vi "Drop Waypoint.vi"(1 "TA Speed":dbl, 2 "TA GPS":cluster{"X pos":i32, "Y pos":i32, "Heading":dbl}={"X pos"=250, "Y pos"=250, "Heading"=0.0}, 3 "Our GPS":cluster{"X pos":i32, "Y pos":i32, "Heading":dbl}={"X pos"=250, "Y pos"=250, "Heading"=0.0}) -> (0 "Output Waypoint":T1={"Type"=enum."Start", "X"=250, "Y"=250, "Speed"=0, "Behaviors"=enum."Open Water Transit"})   [LabVIEW 2014]
panel:
  in  "Waypoint seed":T1={"Type"=enum."Start", "X"=250, "Y"=250, "Speed"=0, "Behaviors"=enum."Open Water Transit"}
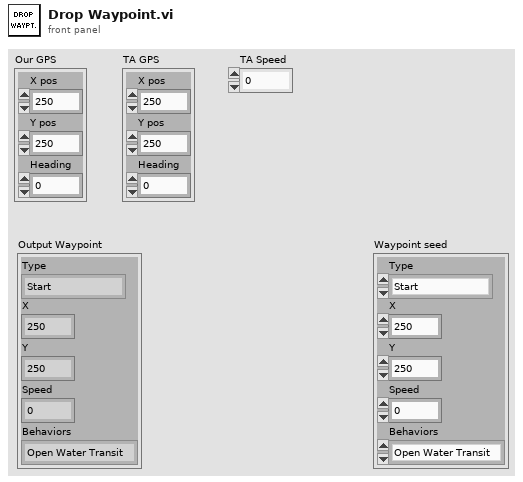
[diagram p1: front panel]
types:
  T1 = cluster{"Type":enum16{"Start", "Waypoint", "End"}, "X":i32, "Y":i32, "Speed":i32, "Behaviors":enum16{"Open Water Transit", "P-Wall Follow", "S-Wall Follow", "Dock", "Chase"}}
  T2 = enum16{"Open Water Transit", "P-Wall Follow", "S-Wall Follow", "Dock", "Chase"}
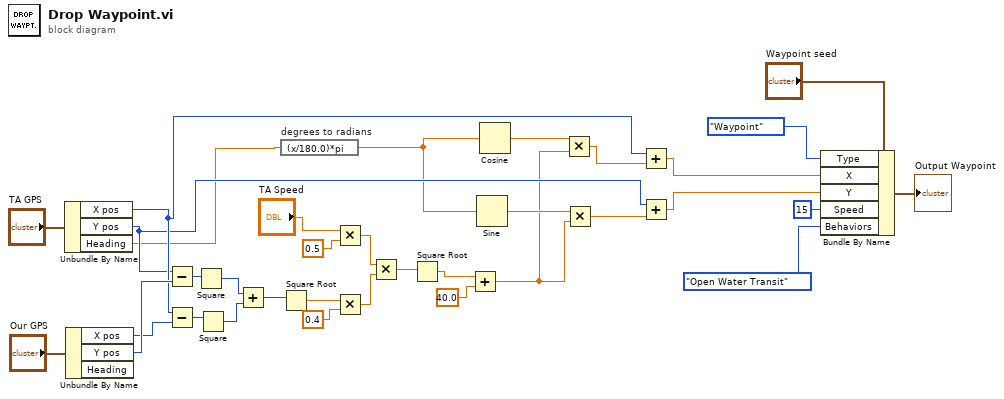
[diagram p0: block diagram]
diagram:
  n1 = Unbundle By Name("TA GPS") -> ("X pos"=w12:i32, "Y pos"=w10:i32, "Heading"=w2:dbl)
  n2 = Unbundle By Name("Our GPS") -> ("X pos"=w27:i32, "Y pos"=w28:i32)  [unwired: 1 out]
  n3 = Subtract(x=w10, y=w28) -> (x-y=w26:i32)
  n4 = Subtract(x=w12, y=w27) -> (x-y=w25:i32)
  n5 = Square(x=w26) -> (x^2=w23:i32)
  n6 = Square(x=w25) -> (x^2=w22:i32)
  n7 = Add(x=w23, y=w22) -> (x+y=w24:i32)
  n8 = expression code="(x/180.0)*pi" "degrees to radians"(w2) -> (w1:dbl)
  n9 = Square Root(x=w24) -> (sqrt(x)=w21:dbl)
  n10 = Multiply(x="TA Speed", y=0.5) -> (x*y=w3:dbl)
  n11 = Multiply(x=w21, y=0.4) -> (x*y=w18:dbl)
  n12 = Multiply(x=w3, y=w18) -> (x*y=w6:dbl)
  n13 = Square Root(x=w6) -> (sqrt(x)=w5:dbl)
  n14 = Add(x=w5, y=40.0) -> (x+y=w8:dbl)
  n15 = Sine(x=w1) -> (sin(x)=w16:dbl)
  n16 = Cosine(x=w1) -> (cos(x)=w15:dbl)
  n17 = Multiply(x=w15, y=w8) -> (x*y=w11:dbl)
  n18 = Multiply(x=w16, y=w8) -> (x*y=w9:dbl)
  n19 = Add(x=w12, y=w11) -> (x+y=w13:dbl)
  n20 = Add(x=w10, y=w9) -> (x+y=w14:dbl)
  n21 = Bundle By Name(cluster="Waypoint seed", "Type"=enum16{"Start", "Waypoint", "End"}."Waypoint", "X"=w13, "Y"=w14, "Speed"=15, "Behaviors"=T2."Open Water Transit") -> (→"Output Waypoint":T1)
